vi "update_progress_bar.vi"(7 "selected":bool, 10 "Numeric":dbl, 11 "Knob in":refnum<vi>) -> (3 "Knob out":refnum<vi>)   [LabVIEW 2015]
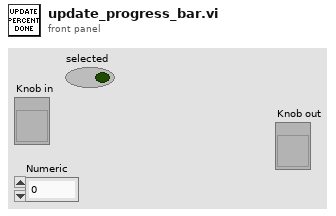
[diagram p1: front panel]
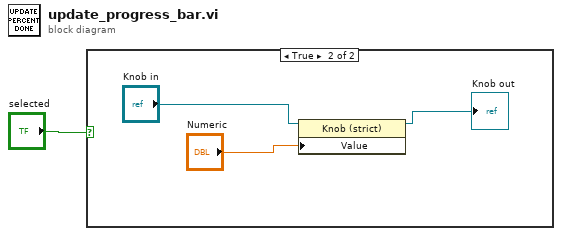
[diagram p0: block diagram]
diagram:
  n1 = case shown="True" "selected" {
    frame False {
    }
    frame True {
      n2 = property class="Knob (strict)"(reference="Knob in", "Value"="Numeric") -> (reference out=→"Knob out":refnum<vi>)  [unwired: 1 in, 1 out]
    }
  }
